vi "数据查询_数据查询.vi"() -> ()   [LabVIEW 2016]
uses:
  <vilib>/Utility/miscctls.llb/LVPointTypeDef.ctl
  <vilib>/addons/database/_DB Variant To Data/Database Variant To Data.xnode
panel:
  in  "触发查询":bool
  out "确定查询":bool
  out "显示项":string[](array[string])
  out "condition":string
  out "Line Chart":T1(xcontrol)
  in  "数据列表选择框":string(xcontrol)
  out "选中数据表":string
  in  "条件筛选":bool
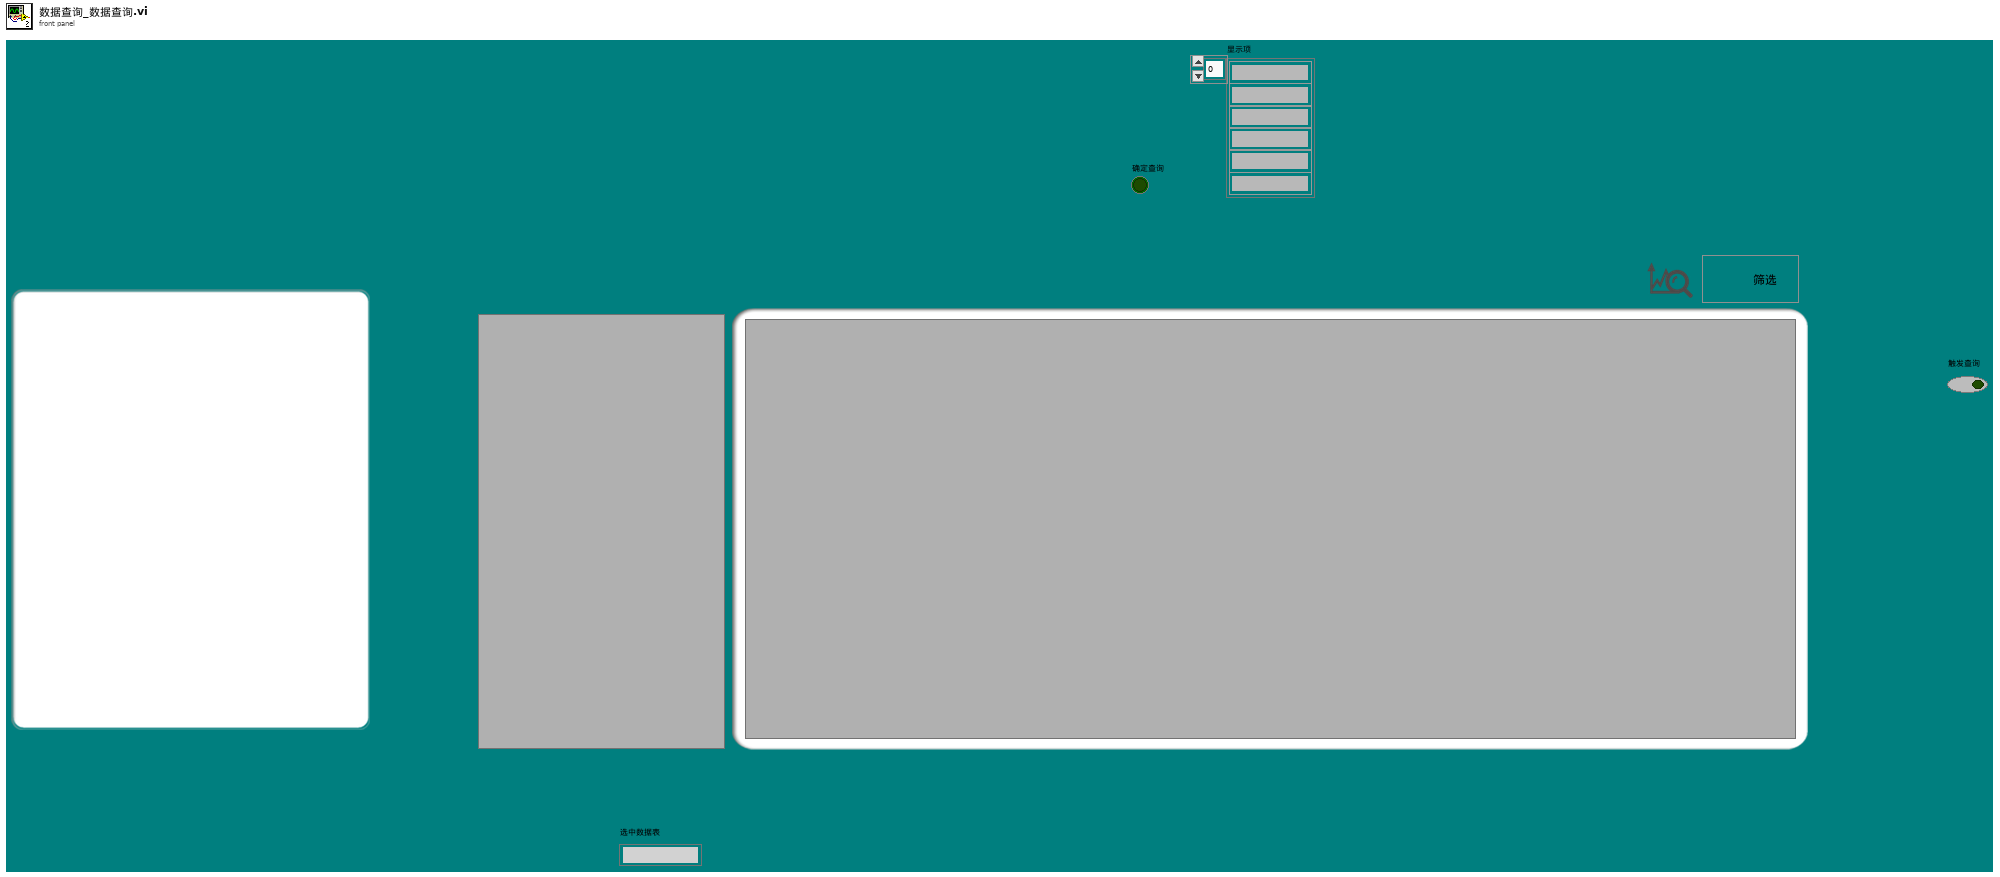
[diagram p1: front panel]
types:
  T1 = cluster{"X-Axis":string[], "Plots":cluster{"Data":dbl[], "Label":string, "Y-Axis":enum16{"Y-Axis 1", "Y-Axis 2", "Y-Axis 3", "Y-Axis 4", "Y-Axis 5", "Y-Axis 6", "Y-Axis 7", "Y-Axis 8", "Y-Axis 9", "Y-Axis 10"}, "Color":u32, "unit":string}[], "Plot Title":string}
  T2 = typedef "LVPointTypeDef.ctl" = cluster{"Horizontal":i16, "Vertical":i16}
  T3 = cluster{"Data":dbl[], "Label":string, "Y-Axis":enum16{"Y-Axis 1", "Y-Axis 2", "Y-Axis 3", "Y-Axis 4", "Y-Axis 5", "Y-Axis 6", "Y-Axis 7", "Y-Axis 8", "Y-Axis 9", "Y-Axis 10"}, "color":u32, "unit":string}
  T4 = cluster{"Data":dbl[], "Label":string, "Y-Axis":enum16{"Y-Axis 1", "Y-Axis 2", "Y-Axis 3", "Y-Axis 4", "Y-Axis 5", "Y-Axis 6", "Y-Axis 7", "Y-Axis 8", "Y-Axis 9", "Y-Axis 10"}, "color":u32, "unit":string}[]
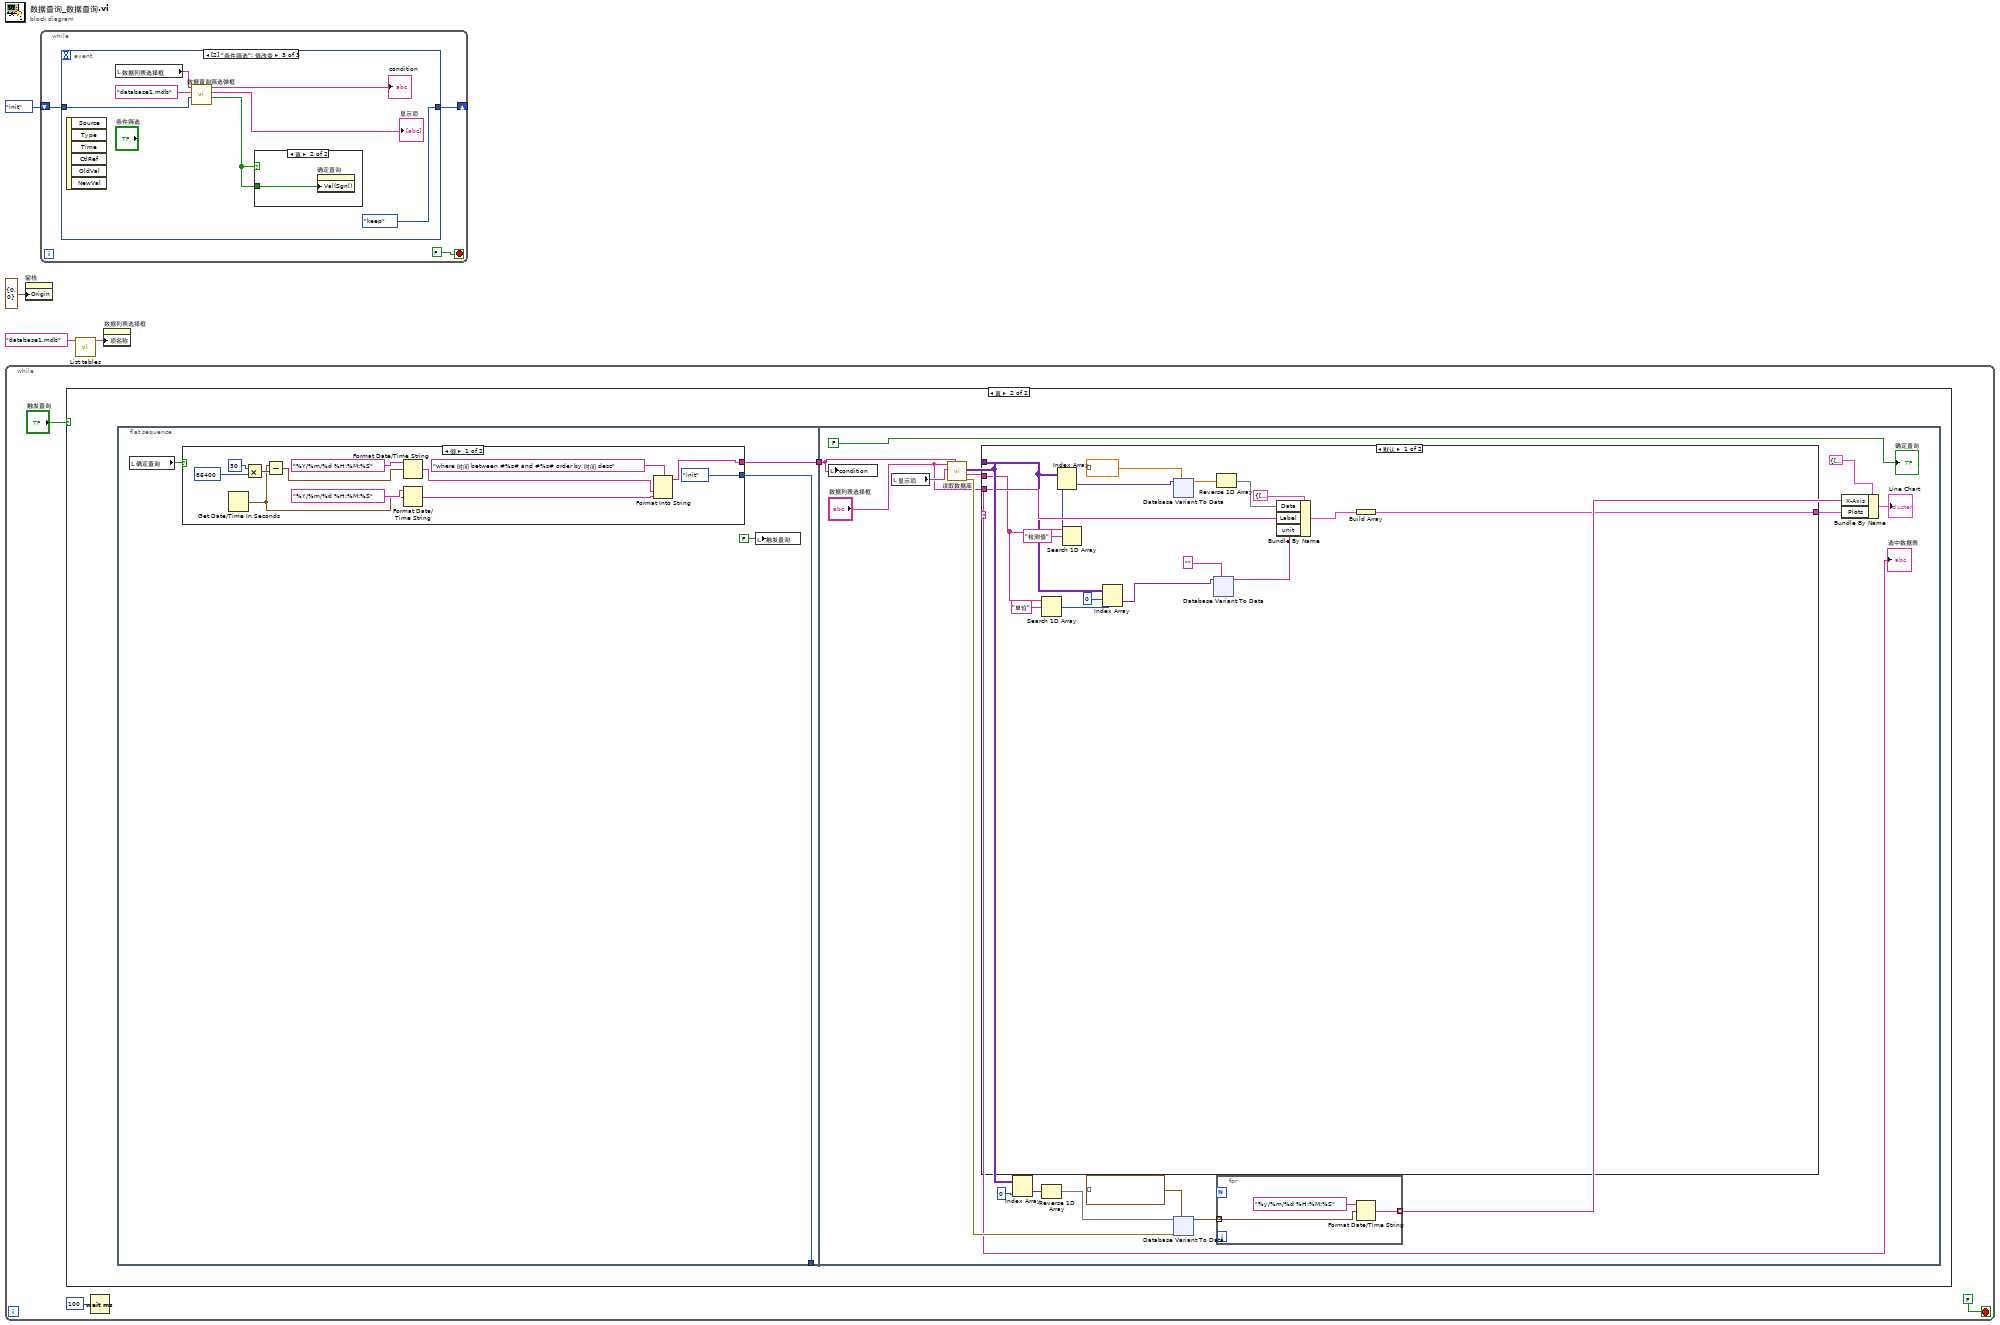
[diagram p0: block diagram]
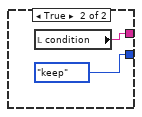
[diagram p3: hidden frame]
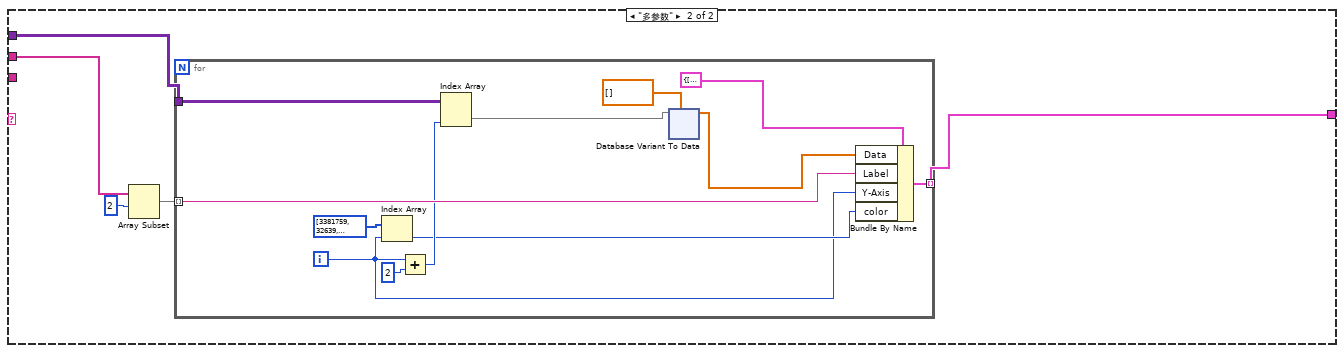
[diagram p4: hidden frame]
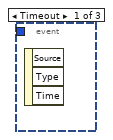
[diagram p5: hidden frame]
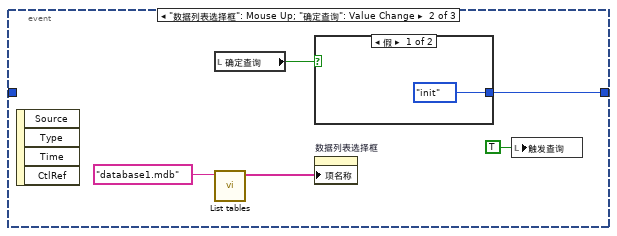
[diagram p6: hidden frame]
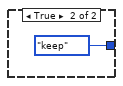
[diagram p7: hidden frame]
diagram:
  n1 = while {
    stop <- FALSE stop-if-true
    n2 = case shown="真" "触发查询" {
      frame False {
      }
      frame True {
        n3 = flat-sequence {
          tunnel: [w11] -> w8
          tunnel: [w10] -> _
          tunnel: w8 -> [w31]
          frame #0 {
            n4 = local read "确定查询"() -> (w12:bool)
            n5 = case shown="假" w12 {
              tunnel: [w15 w25] -> w11
              tunnel: [enum16{"init", "keep"}."init" ("是否初始化") enum16{"init", "keep"}."keep" ("是否初始化")] -> w10
              frame False {
                n6 = Get Date/Time In Seconds() -> (seconds since 1Jan1904=w13:timestamp)
                n7 = Multiply(x=30, y=86400) -> (x*y=w16:i32)
                n8 = Subtract(x=w13, y=w16) -> (x-y=w21:timestamp)
                n9 = Format Date/Time String(time format string (%c)="%Y/%m/%d %H:%M:%S" ("时间格式字符串(%c)"), seconds (now)=w21) -> (date/time string=w23:string)  [unwired: 1 in]
                n10 = Format Date/Time String(time format string (%c)="%Y/%m/%d %H:%M:%S" ("时间格式字符串(%c)"), seconds (now)=w13) -> (date/time string=w24:string)  [unwired: 1 in]
                n11 = Format Into String(format string="where 时间 between #%s# and #%s# order by 时间 desc", w23, w24) -> (resulting string=w15:string)  [unwired: 2 in, 1 out]
              }
              frame True {
                n12 = local read "condition"() -> (w25:string)
              }
            }
            n13 = local write "触发查询"(FALSE ("触发查询")) -> ()
          }
          frame #1 {
            n14 = local write "condition"(w31) -> ()
            n15 = local read "显示项"() -> (w33:string[])
            n16 = call "读取数据库.vi"("condition"=w31, "显示项"=w33, "组合框"="数据列表选择框") -> ("error out"=w39:errorcluster, "columns"=w34:string[], "data"=w38:variant[][])  [unwired: 5 in, 1 out]
            n17 = case shown="默认" "数据列表选择框" {
              tunnel: w38 -> [w47 w135]
              tunnel: [w56 w131] -> w35
              tunnel: "数据列表选择框" -> [w55 _]
              tunnel: w34 -> [w50 w134]
              frame Default {
                n18 = Search 1D Array(1D array=w50, element="单位" ("元素")) -> (index of element=w48:i32)  [unwired: 1 in]
                n19 = Search 1D Array(1D array=w50, element="检测值" ("元素")) -> (index of element=w51:i32)  [unwired: 1 in]
                n20 = Index Array(array=w47, index (col)=w51) -> (element=w60:variant[])  [unwired: 1 in]
                n21 = Index Array(array=w47, index (row)=0 ("禁用的索引 (行)"), index (col)=w48) -> (element=w46:variant)
                n22 = xnode "Database Variant To Data"("database variant"=w60, "type"=sgl[] []) -> ("data"=w58:sgl[])  [unwired: 1 in, 1 out]
                n23 = xnode "Database Variant To Data"("database variant"=w46, "type"="") -> ("data"=w43:string)  [unwired: 1 in, 1 out]
                n24 = Reverse 1D Array(array=w58) -> (reversed array=w53:sgl[])
                n25 = Bundle By Name(cluster=T3 {"Data"=[], "Label"="", "Y-Axis"=enum."Y-Axis 1", "color"=3381759, "unit"=""} ("Plot"), "Data"=w53, "Label"=w55, "unit"=w43) -> (w57:T3)
                n26 = Build Array(w57) -> (w56:T4)
              }
              frame "多参数" {
                n27 = Array Subset(array=w134, index=2 ("索引")) -> (w132:string[])  [unwired: 1 in]
                n28 = for {
                  tunnel: w135 -> [w147]
                  tunnel: [w143] -> w131 mode=indexing
                  tunnel: w132 -> [w142] mode=indexing
                  i -> [w137]
                  n29 = Index Array(array=u32[] [3381759, 32639, 16744576, 16776960, 16711680, 16860, 8388863, 8404992, 10654332, 12819898], index=w137) -> (element=w138:u32)
                  n30 = Add(x=w137, y=2) -> (x+y=w140:i32)
                  n31 = Index Array(array=w147, index (col)=w140) -> (element=w146:variant[])  [unwired: 1 in]
                  n32 = xnode "Database Variant To Data"("database variant"=w146, "type"=sgl[] []) -> ("data"=w144:sgl[])  [unwired: 1 in, 1 out]
                  n33 = Bundle By Name(cluster=T3 {"Data"=[], "Label"="", "Y-Axis"=enum."Y-Axis 1", "color"=3381759, "unit"=""} ("Plot"), "Data"=w144, "Label"=w142, "Y-Axis"=w137, "color"=w138) -> (w143:T3)
                }
              }
            }
            n34 = Index Array(array=w38, index (col)=0 ("禁用的索引 (列)")) -> (element=w41:variant[])  [unwired: 1 in]
            n35 = Reverse 1D Array(array=w41) -> (reversed array=w30:variant[])
            n36 = xnode "Database Variant To Data"("database variant"=w30, "error in (no error)"=w39, "type"=timestamp[] []) -> ("data"=w37:timestamp[])  [unwired: 1 out]
            n37 = for {
              tunnel: w37 -> [w188] mode=indexing
              tunnel: [w187] -> w36 mode=indexing
              n38 = Format Date/Time String(time format string (%c)="%y/%m/%d %H:%M:%S" ("时间格式字符串(%c)"), seconds (now)=w188) -> (date/time string=w187:string)  [unwired: 1 in]
            }
            n39 = Bundle By Name(cluster=T1 {"X-Axis"=[], "Plots"=[], "Plot Title"=""} ("Line Chart"), "X-Axis"=w36, "Plots"=w35) -> (→"Line Chart":T1)
            "选中数据表" <- "数据列表选择框"
            "确定查询" <- FALSE ("确定查询")
          }
        }
      }
    }
    n40 = Wait (ms)(milliseconds to wait=u32 100 ("等待时间（毫秒）")) -> ()  [unwired: 1 out]
  }
  n41 = property on="窗格" class="Pane"("Origin"=T2 {"Horizontal"=0, "Vertical"=0} ("原点")) -> ()  [unwired: 2 in, 2 out]
  n42 = while {
    shift-right: [w241] -> _
    shift-left: enum16{"init", "keep"}."init" ("是否初始化") -> [w242]
    stop <- FALSE stop-if-true
    n43 = event shown="[2] \"条件筛选\": 值改变" {
      selector: _ -> [_ _ _]
      dyn-events: _ -> [_ _ _]
      timeout: _ -> [_ _ _]
      tunnel: w242 -> [_ _ w253]
      tunnel: [_ w245 enum16{"init", "keep"}."keep" ("是否初始化")] -> w241
      event Timeout {
        n44 = event-data() -> ()  [unwired: 1 in, 3 out]
      }
      event "数据列表选择框": Mouse Up; "确定查询": Value Change {
        n45 = event-data() -> ()  [unwired: 1 in, 4 out]
        n46 = local read "确定查询"() -> (w246:bool)
        n47 = call "List tables.vi"("database"="database1.mdb") -> ("tables"=w247:string[])  [unwired: 9 in, 1 out]
        n48 = case shown="假" w246 {
          tunnel: [enum16{"init", "keep"}."init" ("是否初始化") enum16{"init", "keep"}."keep" ("是否初始化")] -> w245
          frame False {
          }
          frame True {
          }
        }
        n49 = property on="数据列表选择框" class="数据列表选择框 (严格)"("项名称"=w247) -> ()  [unwired: 2 in, 2 out]
        n50 = local write "触发查询"(TRUE ("触发查询")) -> ()
      }
      event "条件筛选": Value Change {
        n51 = event-data() -> ()  [unwired: 1 in, 6 out]
        n52 = local read "数据列表选择框"() -> (w255:string)
        n53 = call "数据查询筛选弹框.vi"("是否初始化"=w253, "database"="database1.mdb", "table"=w255) -> ("确定输出"=w252:bool, "显示项"=→"显示项":string[], "condition"=→"condition":string)  [unwired: 5 in, 1 out]
        n54 = case shown="真" w252 {
          tunnel: w252 -> [_ w258]
          frame False {
          }
          frame True {
            n55 = property on="确定查询" class="Bool (严格)"("Val(Sgnl)"=w258) -> ()  [unwired: 2 in, 2 out]
          }
        }
      }
    }
  }
  n56 = call "List tables.vi"("database"="database1.mdb") -> ("tables"=w2:string[])  [unwired: 9 in, 1 out]
  n57 = property on="数据列表选择框" class="数据列表选择框 (严格)"("项名称"=w2) -> ()  [unwired: 2 in, 2 out]
